vi "Test Client AMQPAsync.vi"() -> ()   [LabVIEW 2019, in "BNT_SLMsgLogger.lvlib"]
doc: "Synchronously sends messages to and receives messages from the Client VI using the Skyline Message API."
uses:
  BNT_SLMsgLogger.lvlib
  <vilib>/Skyline/Message/AMQP/async/Open (Async).vi
  <vilib>/Skyline/Message/AMQP/NI Skyline Message AMQP (Async).lvclass
  <vilib>/Skyline/Message/NI Skyline Message.lvclass
panel:
  in  "Clear":bool
  out "Received Message":string
  # "Overview: Demonstrates the use of the SystemLink Message functions to asynchronously receive messages\n.Requirements: LabVIEW Base Development System\n                            SystemLink API\nInstructions:\n1. Ensure the server is running locally or the system running this VI is managed by the server.\n2. Run the VI either on the host or on a Real-Time target.\n3. Open the block diagram an choose topic to subscribe.\n4. Run the Host VI if it isn't running already.\n4. Watch the Received Message field to watch for messages received from the Host."
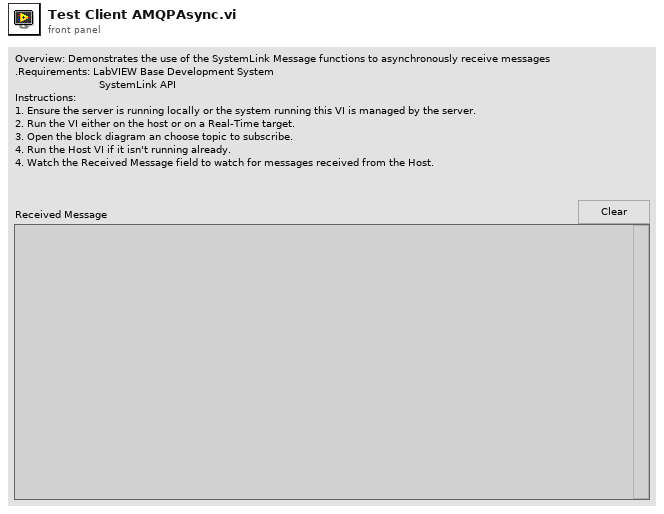
[diagram p1: front panel]
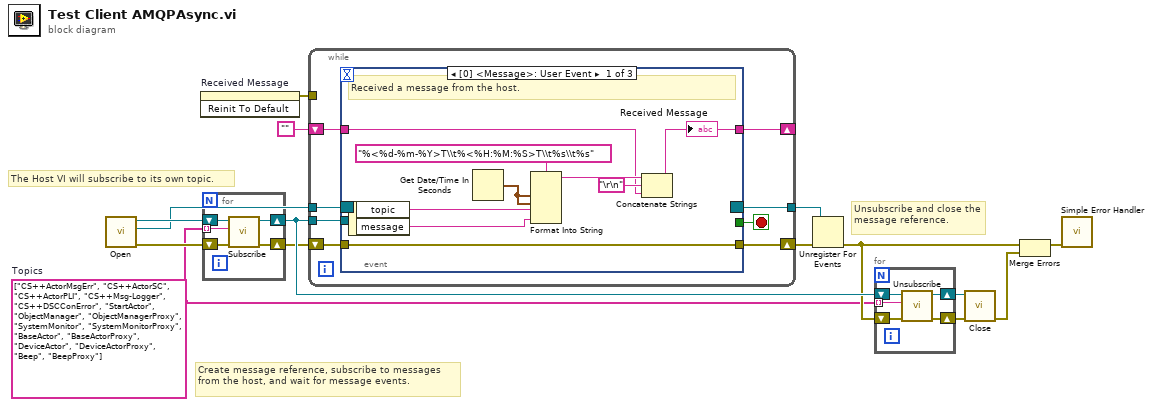
[diagram p0: block diagram]
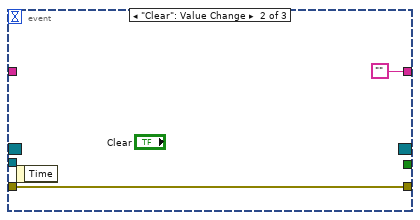
[diagram p2: hidden frame]
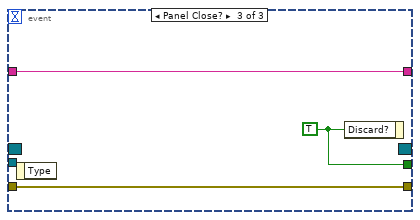
[diagram p3: hidden frame]
diagram:
  w2 = string[] ["CS++ActorMsgErr", "CS++ActorSC", "CS++ActorPLI", "CS++Msg-Logger", "CS++DSCConError", "StartActor", "ObjectManager", "ObjectManagerProxy", "SystemMonitor", "SystemMonitorProxy", "BaseActor", "BaseActorProxy", "DeviceActor", "DeviceActorProxy", "Beep", "BeepProxy"]  # Topics
  # "The Host VI will subscribe to its own topic."
  # "Unsubscribe and close the message reference."
  # "Create message reference, subscribe to messages from the host, and wait for message events."
  n1 = call-poly <vilib>:"Open.vi"() -> ("error out"=w13:errorcluster, "event registration refnum"=w4:refnum<event-registration>, "message session"=w14:refnum<class "NI Skyline Message AMQP (Async).lvclass">)  [unwired: 9 in]
  n2 = invoke on="Received Message" class="Str" method="Reinit To Default"() -> (error out=w12:errorcluster)  [unwired: 3 in, 2 out]
  n3 = for {
    tunnel: w2 -> [w16] mode=indexing
    shift-right: [w18] -> w7
    shift-left: w14 -> [w20]
    shift-right: [w17] -> w6
    shift-left: w13 -> [w19]
    n4 = call-dynamic "Subscribe.vi"("error in (no error)"=w19, "topic"=w16, "message session in"=w20) -> ("error out"=w17:errorcluster, "message session out"=w18:refnum<class "NI Skyline Message AMQP (Async).lvclass">)  [unwired: 7 in]
  }
  n5 = while {
    tunnel: [w26] -> w5
    shift-right: [w23] -> w15
    shift-left: w6 -> [w28]
    tunnel: w12 -> [_]
    tunnel: w7 -> [w25]
    tunnel: w4 -> [w24]
    shift-right: [w21] -> _
    shift-left: "" -> [w22]
    stop <- w27 stop-if-true
    n6 = event shown="[0] <Message>: User Event" {
      selector: w24 -> [_ _ _]
      dyn-events: [_ _ _] -> w26
      timeout: _ -> [_ _ _]
      tunnel: w28 -> [w37 w39 w41]
      tunnel: [_ _ w42] -> w27
      tunnel: w25 -> [_ _ _]
      tunnel: [w37 w39 w41] -> w23
      tunnel: w22 -> [w29 _ w40]
      tunnel: [w32 "" w40] -> w21
      event User Event {
        # "Received a message from the host."
        n7 = event-data() -> ("topic"=w34:string, "message"=w33:string)  [unwired: 1 in]
        n8 = Get Date/Time In Seconds() -> (seconds since 1Jan1904=w35:timestamp)
        n9 = Format Into String(format string="%<%d-%m-%Y>T\\t%<%H:%M:%S>T\\t%s\\t%s", w35, w35, w34, w33) -> (resulting string=w31:string)  [unwired: 2 in, 1 out]
        n10 = Concatenate Strings(w31, "\r\n", w29) -> (w32:string)
        "Received Message" <- w32
      }
      event "Clear": Value Change {
        n11 = event-data() -> ()  [unwired: 1 in, 1 out]
      }
      event Panel Close? {
        w42 = TRUE ("Discard?")
        n12 = event-data() -> ()  [unwired: 1 in, 1 out]
        n13 = event-data("Discard?"=w42) -> ()  [unwired: 1 in, 1 out]
      }
    }
  }
  n14 = Unregister For Events(event registration refnum=w5, error in=w15) -> (error out=w3:errorcluster)
  n15 = for {
    tunnel: w2 -> [w43] mode=indexing
    shift-right: [w46] -> w10
    shift-left: w7 -> [w45]
    shift-right: [w47] -> w11
    shift-left: w3 -> [w44]
    n16 = call-dynamic "Unsubscribe.vi"("error in (no error)"=w44, "topic"=w43, "message session in"=w45) -> ("error out"=w47:errorcluster, "message session out"=w46:refnum<class "NI Skyline Message AMQP (Async).lvclass">)  [unwired: 7 in]
  }
  n17 = call-dynamic "Close.vi"("error in (no error)"=w11, "message session"=w10) -> ("error out"=w8:errorcluster)  [unwired: 9 in]
  n18 = Merge Errors(w3, w8) -> (w9:errorcluster)
  n19 = call <vilib>:"Simple Error Handler.vi"("error in (no error)"=w9) -> ()  [unwired: 4 in, 5 out]
